vi "get_type.vi"(11 "Cluster":variant) -> (3 "types":u8[](array[numeric]))   [LabVIEW 2012]
uses:
  <userlib>/_OpenG.lib/lvdata/lvdata.llb/Type Descriptor Enumeration__ogtk.ctl
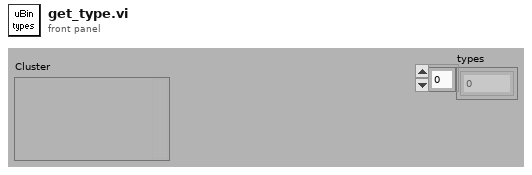
[diagram p1: front panel]
types:
  T1 = typedef "Type Descriptor Enumeration__ogtk.ctl" = enum8{"<Null>", "I8", "I16", "I32", "I64", "U8", "U16", "U32", "U64", "SGL", "DBL", "EXT", "CSG", "CDB", "CXT", "0x0F", "0x10", "0x11", "0x12", "0x13", "0x14", "Enum U8", "Enum U16", "Enum U32", "Enum U64", "SGL PQ", "DBL PQ", "EXT PQ", "CSG PQ", "CDB PQ", "CXT PQ", "0x1F", "0x20", "Boolean", "0x22", "0x23", "0x24", "0x25", "0x26", "0x27", "0x28", "0x29", "0x2A", "0x2B", "0x2C", "0x2D", "0x2E", "0x2F", "String", "0x31", "Path", "Pict", "0x34", "0x35", "0x36", "DAQ", "0x38", "0x39", "0x3A", "0x3B", "0x3C", "0x3D", "0x3E", "0x3F", "Array", "0x41", "0x42", "0x43", "0x44", "0x45", "0x46", "0x47", "0x48", "0x49", "0x4A", "0x4B", "0x4C", "0x4D", "0x4E", "0x4F", "Cluster", "0x51", "0x52", "Variant", "Waveform", "0x55", "0x56", "0x57", "0x58", "0x59", "0x5A", "0x5B", "0x5C", "0x5D", "0x5E", "0x5F", "0x60", "0x61", "0x62", "0x63", "0x64", "0x65", "0x66", "0x67", "0x68", "0x69", "0x6A", "0x6B", "0x6C", "0x6D", "0x6E", "0x6F", "Refnum"}
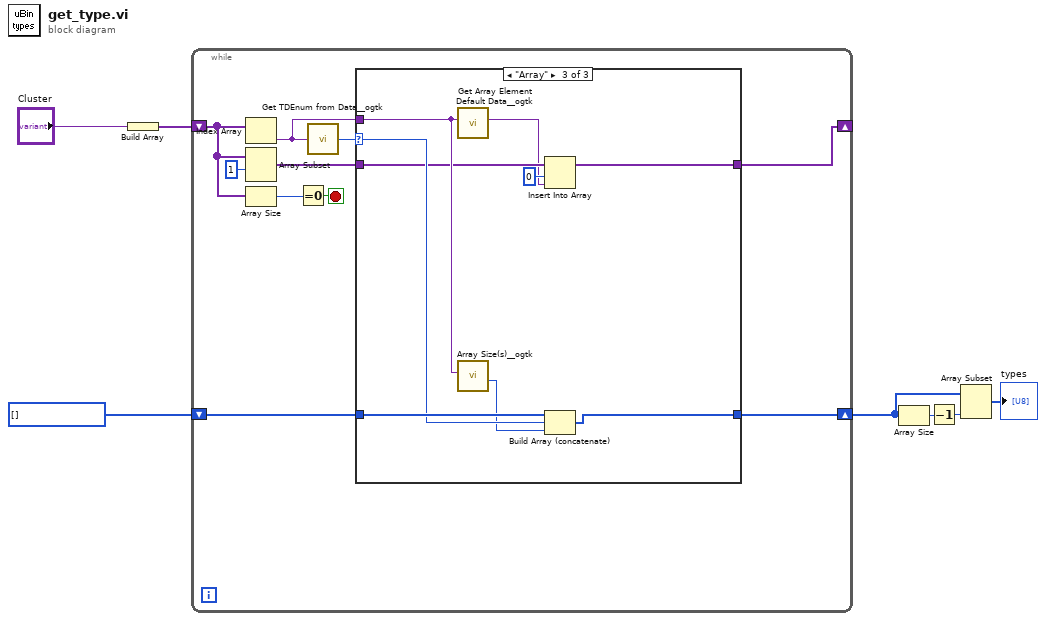
[diagram p0: block diagram]
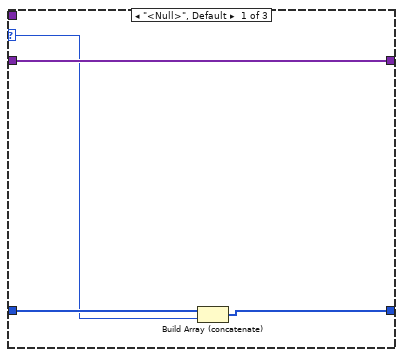
[diagram p2: hidden frame]
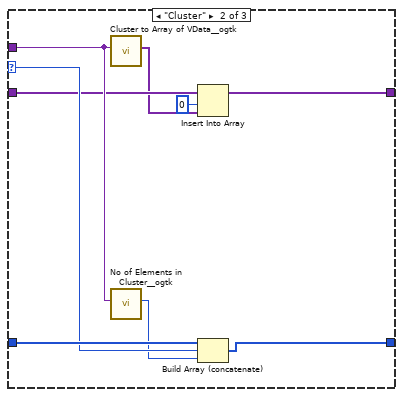
[diagram p3: hidden frame]
diagram:
  w4 = T1[] [] items=["<Null>", "I8", "I16", "I32", "I64", "U8", "U16", "U32", "U64", "SGL", "DBL", "EXT", "CSG", "CDB", "CXT", "0x0F", "0x10", "0x11", "0x12", "0x13", "0x14", "Enum U8", "Enum U16", "Enum U32", "Enum U64", "SGL PQ", "DBL PQ", "EXT PQ", "CSG PQ", "CDB PQ", "CXT PQ", "0x1F", "0x20", "Boolean", "0x22", "0x23", "0x24", "0x25", "0x26", "0x27", "0x28", "0x29", "0x2A", "0x2B", "0x2C", "0x2D", "0x2E", "0x2F", "String", "0x31", "Path", "Pict", "0x34", "0x35", "0x36", "DAQ", "0x38", "0x39", "0x3A", "0x3B", "0x3C", "0x3D", "0x3E", "0x3F", "Array", "0x41", "0x42", "0x43", "0x44", "0x45", "0x46", "0x47", "0x48", "0x49", "0x4A", "0x4B", "0x4C", "0x4D", "0x4E", "0x4F", "Cluster", "0x51", "0x52", "Variant", "Waveform", "0x55", "0x56", "0x57", "0x58", "0x59", "0x5A", "0x5B", "0x5C", "0x5D", "0x5E", "0x5F", "0x60", "0x61", "0x62", "0x63", "0x64", "0x65", "0x66", "0x67", "0x68", "0x69", "0x6A", "0x6B", "0x6C", "0x6D", "0x6E", "0x6F", "Refnum"]
  n1 = Build Array("Cluster") -> (w3:variant[])
  n2 = while {
    shift-right: [w16] -> _
    shift-left: w3 -> [w12]
    shift-right: [w13] -> w5
    shift-left: w4 -> [w14]
    stop <- w11 stop-if-true
    n3 = Index Array(array=w12) -> (element=w8:variant)  [unwired: 1 in]
    n4 = Array Subset(array=w12, index=1) -> (w15:variant[])  [unwired: 1 in]
    n5 = Array Size(array=w12) -> (size(s)=w9:i32)
    n6 = Equal To 0?(x=w9) -> (x = 0?=w11:bool)
    n7 = call <userlib>:"Get TDEnum from Data__ogtk.vi"("Data"=w8) -> ("Type Descriptor Enumeration"=w10:T1)  [unwired: 4 in]
    n8 = case shown="\"Array\"" w10 {
      selector: w10 -> [w18 w28 w37]
      tunnel: [w21 w23 w33] -> w16
      tunnel: w15 -> [w21 w25 w34]
      tunnel: w14 -> [w20 w30 w39]
      tunnel: [w19 w29 w38] -> w13
      tunnel: w8 -> [_ w26 w35]
      frame "<Null>", Default {
        n9 = Build Array (concatenate)(w20, w18) -> (w19:u32[])
      }
      frame "Cluster" {
        n10 = call <userlib>:"Cluster to Array of VData__ogtk.vi"("Cluster"=w26) -> ("Array of VData"=w24:variant[])  [unwired: 9 in, 1 out]
        n11 = call <userlib>:"No of Elements in Cluster__ogtk.vi"("Cluster"=w26) -> ("Number of Elements"=w27:u16)  [unwired: 9 in, 1 out]
        n12 = Insert Into Array(array=w25, index=0, new element=w24) -> (w23:variant[])
        n13 = Build Array (concatenate)(w30, w28, w27) -> (w29:u32[])
      }
      frame "Array" {
        n14 = call <userlib>:"Get Array Element Default Data__ogtk.vi"("Array"=w35) -> ("Array Element Default Data"=w31:variant)  [unwired: 9 in, 1 out]
        n15 = call <userlib>:"Array Size(s)__ogtk.vi"("Array"=w35) -> ("N dims"=w36:u32)  [unwired: 8 in, 2 out]
        n16 = Insert Into Array(array=w34, index=0, new element=w31) -> (w33:variant[])
        n17 = Build Array (concatenate)(w39, w37, w36) -> (w38:u32[])
      }
    }
  }
  n18 = Array Size(array=w5) -> (size(s)=w7:i32)
  n19 = Decrement(x=w7) -> (x-1=w6:i32)
  n20 = Array Subset(array=w5, length=w6) -> (→"types":u32[])  [unwired: 1 in]
